vi "Create Main Message Queues.vi"(8 "error in (no error)":errorcluster, 11 "Process Name":string="Feed Module 1") -> (0 "error out":errorcluster, 3 "Message Queues out":T1)   [LabVIEW 2021]
doc: "This VI creates and initializes all the message queues for your application. If your application requires more than one message queue, right-click the \"Message Queues\" constant above and select Open Type Def. Add the new Message Queue(s) to the type definition, then initialize them in this VI."
uses:
  Main Queue Cluster.ctl
  support/Message Queue/Message Cluster.ctl
  support/Message Queue/Enqueue Message (Single).vi
  support/Message Queue/Message Queue.lvlib
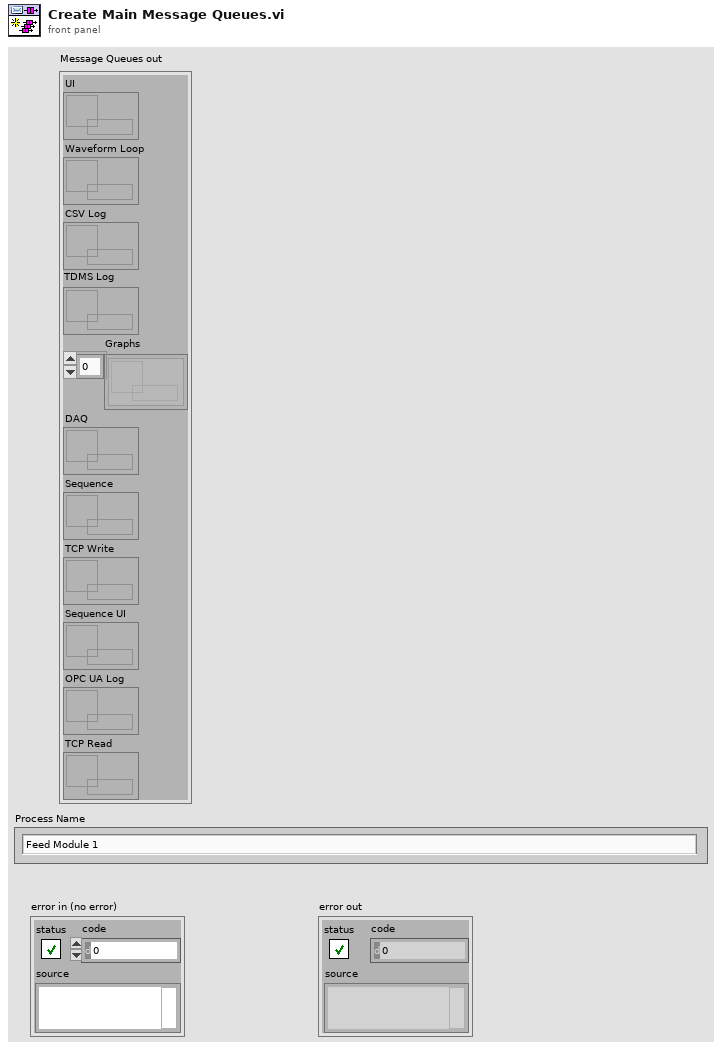
[diagram p1: front panel]
types:
  T1 = typedef "Main Queue Cluster.ctl" = cluster{"UI":refnum<queue>, "Waveform Loop":refnum<queue>, "CSV Log":refnum<queue>, "TDMS Log":refnum<queue>, "Graphs":refnum<queue>[], "DAQ":refnum<queue>, "Sequence":refnum<queue>, "TCP Write":refnum<queue>, "Sequence UI":refnum<queue>, "OPC UA Log":refnum<queue>, "TCP Read":refnum<queue>}
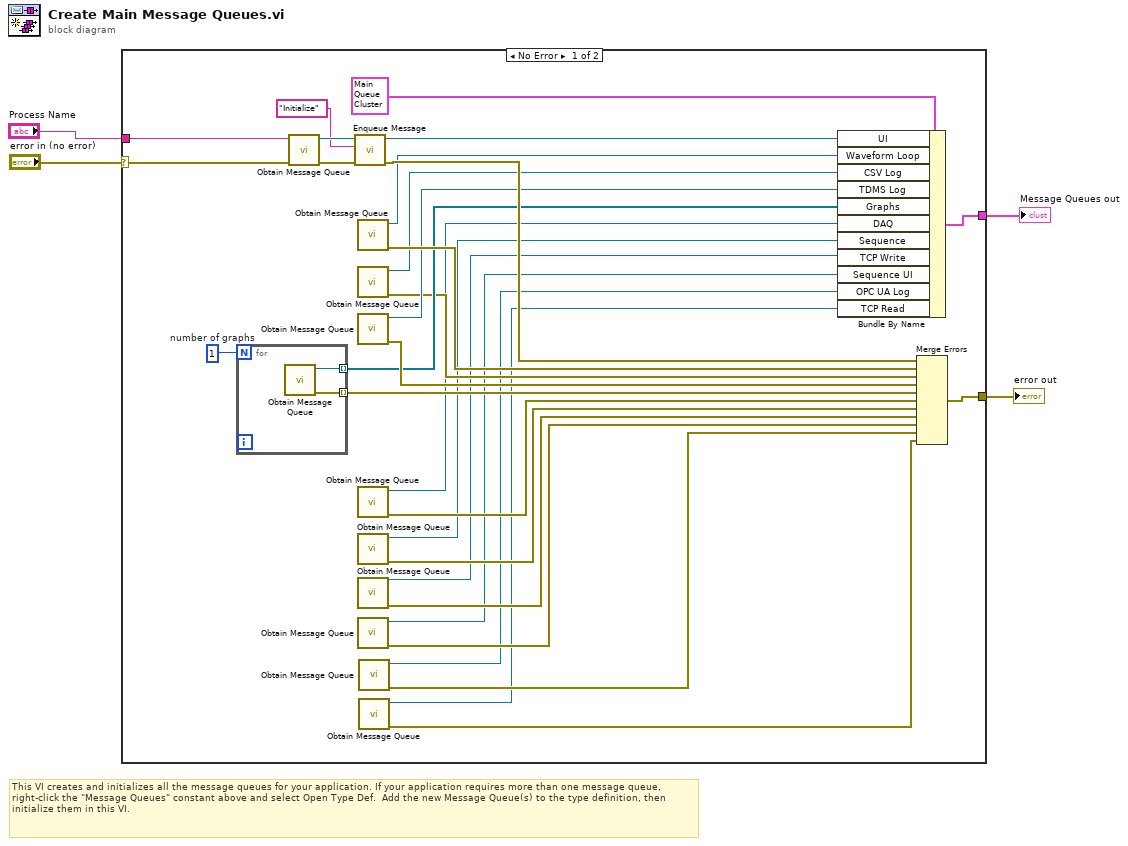
[diagram p0: block diagram]
diagram:
  # "This VI creates and initializes all the message queues for your application. If your application requires more than one message queue, right-click the \"Message Queues\" constant above and select Open Type Def.  Add the new Message Queue(s) to the type definition, then initialize them in this VI."
  n1 = case shown="No Error" "error in (no error)" {
    selector: "error in (no error)" -> [w29 w38]
    tunnel: [w30 w38] -> w4
    tunnel: [w34 _] -> w3
    tunnel: "Process Name" -> [w28 _]
    frame No Error {
      w21 = 1  # number of graphs
      n2 = for {
        N: w21 -> [_]
        tunnel: [w37] -> w20 mode=indexing
        tunnel: [w36] -> w19 mode=indexing
        n3 = call "Obtain Message Queue.vi"() -> ("error out"=w36:errorcluster, "Message Queue"=w37:refnum<queue>)  [unwired: 10 in]
      }
      n4 = call "Obtain Message Queue.vi"("error in (no error)"=w29, "name (unnamed)"=w28) -> ("error out"=w33:errorcluster, "Message Queue"=w32:refnum<queue>)  [unwired: 8 in]
      n5 = call-poly "Enqueue Message.vi"("error in (no error)"=w33, "Message"="Initialize", "Message Queue"=w32) -> ("error out"=w35:errorcluster, "dup Message Queue"=w31:refnum<queue>)  [unwired: 7 in]
      n6 = call "Obtain Message Queue.vi"() -> ("error out"=w24:errorcluster, "Message Queue"=w25:refnum<queue>)  [unwired: 10 in]
      n7 = call "Obtain Message Queue.vi"() -> ("error out"=w17:errorcluster, "Message Queue"=w18:refnum<queue>)  [unwired: 10 in]
      n8 = call "Obtain Message Queue.vi"() -> ("error out"=w23:errorcluster, "Message Queue"=w22:refnum<queue>)  [unwired: 10 in]
      n9 = call "Obtain Message Queue.vi"() -> ("error out"=w15:errorcluster, "Message Queue"=w16:refnum<queue>)  [unwired: 10 in]
      n10 = call "Obtain Message Queue.vi"() -> ("error out"=w13:errorcluster, "Message Queue"=w14:refnum<queue>)  [unwired: 10 in]
      n11 = call "Obtain Message Queue.vi"() -> ("error out"=w11:errorcluster, "Message Queue"=w12:refnum<queue>)  [unwired: 10 in]
      n12 = call "Obtain Message Queue.vi"() -> ("error out"=w9:errorcluster, "Message Queue"=w10:refnum<queue>)  [unwired: 10 in]
      n13 = call "Obtain Message Queue.vi"() -> ("error out"=w7:errorcluster, "Message Queue"=w8:refnum<queue>)  [unwired: 10 in]
      n14 = call "Obtain Message Queue.vi"() -> ("error out"=w6:errorcluster, "Message Queue"=w5:refnum<queue>)  [unwired: 10 in]
      n15 = Bundle By Name(cluster=T1 {"UI"=refnum, "Waveform Loop"=refnum, "CSV Log"=refnum, "TDMS Log"=refnum, "Graphs"=[], "DAQ"=refnum, "Sequence"=refnum, "TCP Write"=refnum, "Sequence UI"=refnum, "OPC UA Log"=refnum, "TCP Read"=refnum} ("Message Queues out"), "UI"=w31, "Waveform Loop"=w25, "CSV Log"=w18, "TDMS Log"=w22, "Graphs"=w20, "DAQ"=w16, "Sequence"=w14, "TCP Write"=w12, "Sequence UI"=w10, "OPC UA Log"=w8, "TCP Read"=w5) -> (w34:T1)
      n16 = Merge Errors(w35, w24, w17, w23, w19, w15, w13, w11, w9, w7, w6) -> (w30:errorcluster)
    }
    frame Error {
    }
  }
  "Message Queues out" <- w3
  "error out" <- w4
